vi "Tag_PID_Param Controls_VIG.vi"(7 "Operation":enum16{"get data", "set data", "initialize"}(ring)=enum."set data", 8 "error in":errorcluster, 10 "tag_ctrl_ref_in":refnum<vi>[](array[refnum]), 11 "tag_data_in":dbl[](array[numeric])) -> (0 "error out":errorcluster, 3 "tag_data_out":dbl[](array[numeric]))   [LabVIEW 2018]
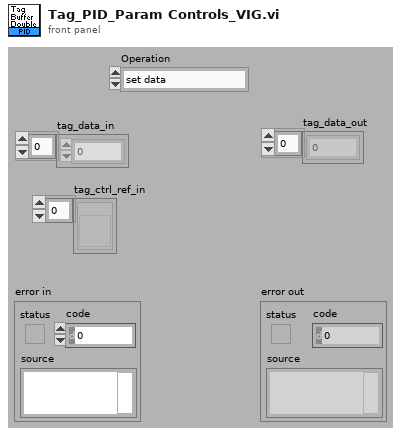
[diagram p1: front panel]
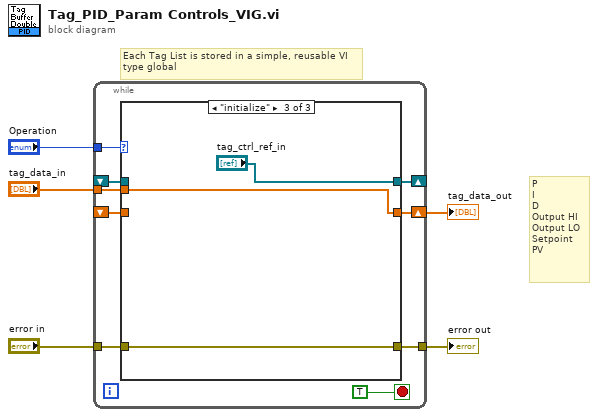
[diagram p0: block diagram]
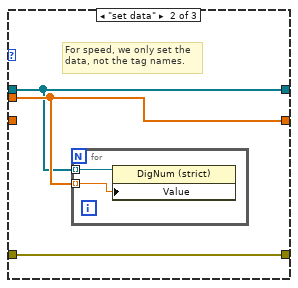
[diagram p3: hidden frame]
diagram:
  # "P\nI\nD\nOutput HI\nOutput LO\nSetpoint\nPV"
  # "Each Tag List is stored in a simple, reusable VI\ntype global"
  n1 = while {
    tunnel: "Operation" -> [w14]
    shift-right: [w12] -> w3
    shift-left: _ -> [w10]
    tunnel: "tag_data_in" -> [w11]
    tunnel: "error in" -> [w9]
    tunnel: [w8] -> w1
    shift-right: [w7] -> _
    shift-left: _ -> [w6]
    stop <- TRUE stop-if-true
    n2 = case shown="\"initialize\"" w14 {
      tunnel: [w17 w19 w23] -> w12
      tunnel: w11 -> [_ w19 w23]
      tunnel: w10 -> [w17 _ _]
      tunnel: w9 -> [w16 w20 w25]
      tunnel: [w16 w20 w25] -> w8
      tunnel: [w15 w18 "tag_ctrl_ref_in"] -> w7
      tunnel: w6 -> [w15 w18 _]
      frame "get data", Default {
      }
      frame "set data" {
        # "For speed, we only set the\ndata, not the tag names."
        n3 = for {
          tunnel: w18 -> [w22] mode=indexing
          tunnel: w19 -> [w21] mode=indexing
          n4 = property class="DigNum (strict)"(reference=w22, "Value"=w21) -> ()  [unwired: 1 in, 2 out]
        }
      }
      frame "initialize" {
      }
    }
  }
  "error out" <- w1
  "tag_data_out" <- w3
